vi "PQ Example INSERT.vi"() -> ()   [LabVIEW 2015]
uses:
  Connection/Single Command (No results).vi
  Connection/PQ Connection.lvclass
panel:
  out "error out":errorcluster
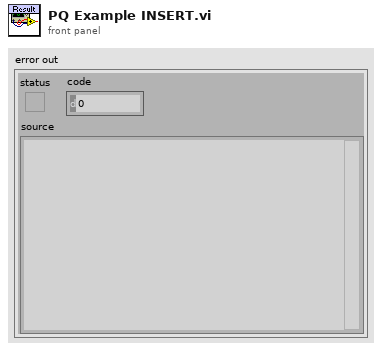
[diagram p1: front panel]
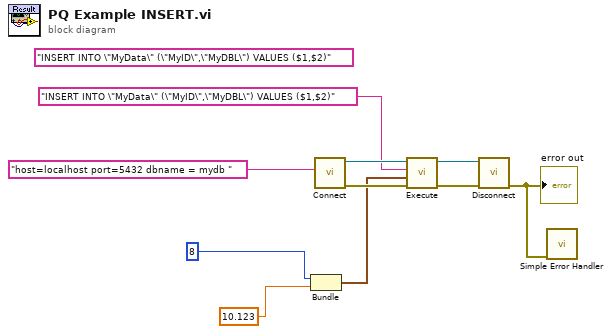
[diagram p0: block diagram]
diagram:
  (unwired) "INSERT INTO \"MyData\" (\"MyID\",\"MyDBL\") VALUES ($1,$2)" ("command")
  n1 = Bundle(8, 10.123) -> (w3:cluster{i32, dbl})  [unwired: 1 in]
  n2 = call "Connect.vi"("conninfo"="host=localhost port=5432 dbname = mydb ") -> ("error out"=w7:errorcluster, "PQ Connection out"=w9:refnum<class "PQ Connection.lvclass">)  [unwired: 9 in]
  n3 = call-poly "Execute.vi"("error in (no error)"=w7, "Variant (Cluster, Array,..)"=w3, "SQL (Single Command)"="INSERT INTO \"MyData\" (\"MyID\",\"MyDBL\") VALUES ($1,$2)" ("command"), "PQ Connection in"=w9) -> ("error out"=w5:errorcluster, "PQ Connection out"=w8:refnum<class "PQ Connection.lvclass">)  [unwired: 6 in]
  n4 = call "Disconnect.vi"("error in (no error)"=w5, "PQ Connection in"=w8) -> ("error out"=w2:errorcluster)  [unwired: 9 in]
  "error out" <- w2
  n5 = call <vilib>:"Simple Error Handler.vi"("error in (no error)"=w2) -> ()  [unwired: 4 in, 5 out]
